vi "Set Response FIFO.vi"(10 "Response FIFO":T1, 11 "Interface in":refnum<class "Engine Interface.lvclass">) -> (3 "Interface out":refnum<class "Engine Interface.lvclass">)   [LabVIEW 2017, in "Data Sharing Framework Engine.lvlib" / "Engine Interface.lvclass"]
uses:
  Engine Interface.lvclass
  16B RT FIFO Reference.ctl
  16B Data.ctl
  16B Payload.ctl
  Engine Interface.lvclass/Engine Interface.ctl
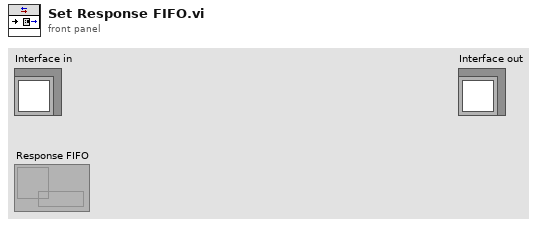
[diagram p1: front panel]
types:
  T1 = typedef "Data Sharing Framework Engine.lvlib/Engine Interface.lvclass/16B RT FIFO Reference.ctl" = refnum<k33>
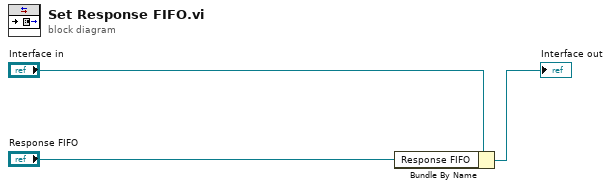
[diagram p0: block diagram]
diagram:
  n1 = Bundle By Name(cluster="Interface in", "Response FIFO"="Response FIFO") -> (→"Interface out":refnum<class "Engine Interface.lvclass">)
